vi "main.vi"() -> ()   [LabVIEW 2022 SP3]
uses:
  controls/State_control.ctl
  controls/Data.ctl
  <vilib>/Utility/TDMS File Viewer/NI_TDMS File Viewer.lvlib
panel:
  out "Current":dbl(graph)
  out "Voltage":dbl(graph)
  out "Current":dbl[](array[numeric])
  out "Voltage":dbl[](array[numeric])
  in  "Pocet prumer":i8 min=1 max=20 step=1
  out "Doba mereni [ms]":i16
  in  "Pocet vz":i32
  in  "vzorky/s":enum16{"Slow", "2F2F"}(ring)
  out "IDN commnad 4":string
  in  "GPD-3303S":refnum<visa-resource-name>
  in  "Stop":bool
  in  "Store data":bool
  in  "Reset array":bool
  in  "Start meas":bool
  out "IDN commnad":string
  in  "Agilent 34401A":refnum<visa-resource-name>
  in  "Agilent 34450A":refnum<visa-resource-name>
  out "IDN commnad 3":string
  out "State":T1=enum."SaveData"
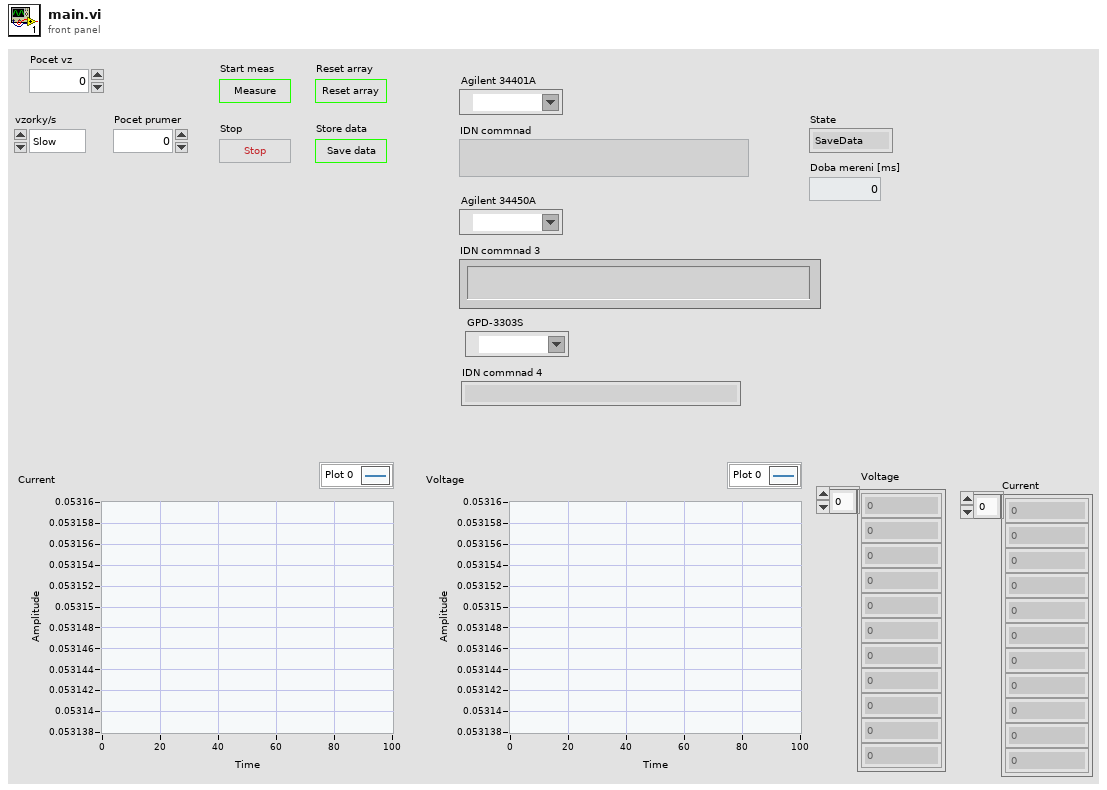
[diagram p1: front panel]
types:
  T1 = typedef "State_control.ctl" = enum16{"Init", "Waiting", "Measure", "SaveData", "Finish"}
  T2 = typedef "Data.ctl" = cluster{"No Sample":i32, "Samples/s":i32, "No to avg":i32, "Voltage":dbl[], "Current":dbl[], "Resistance":dbl[], "Temperature":dbl[], "Avg Voltage":dbl[], "Timestamp":timestamp[], "Avg Current":dbl[]}
  T3 = enum16{"open", "open or create", "create or replace", "create", "open (read-only)"}
  T4 = cluster{"Agilent 34401A":refnum<visa-resource-name>, "Agilent 34450A":refnum<visa-resource-name>}
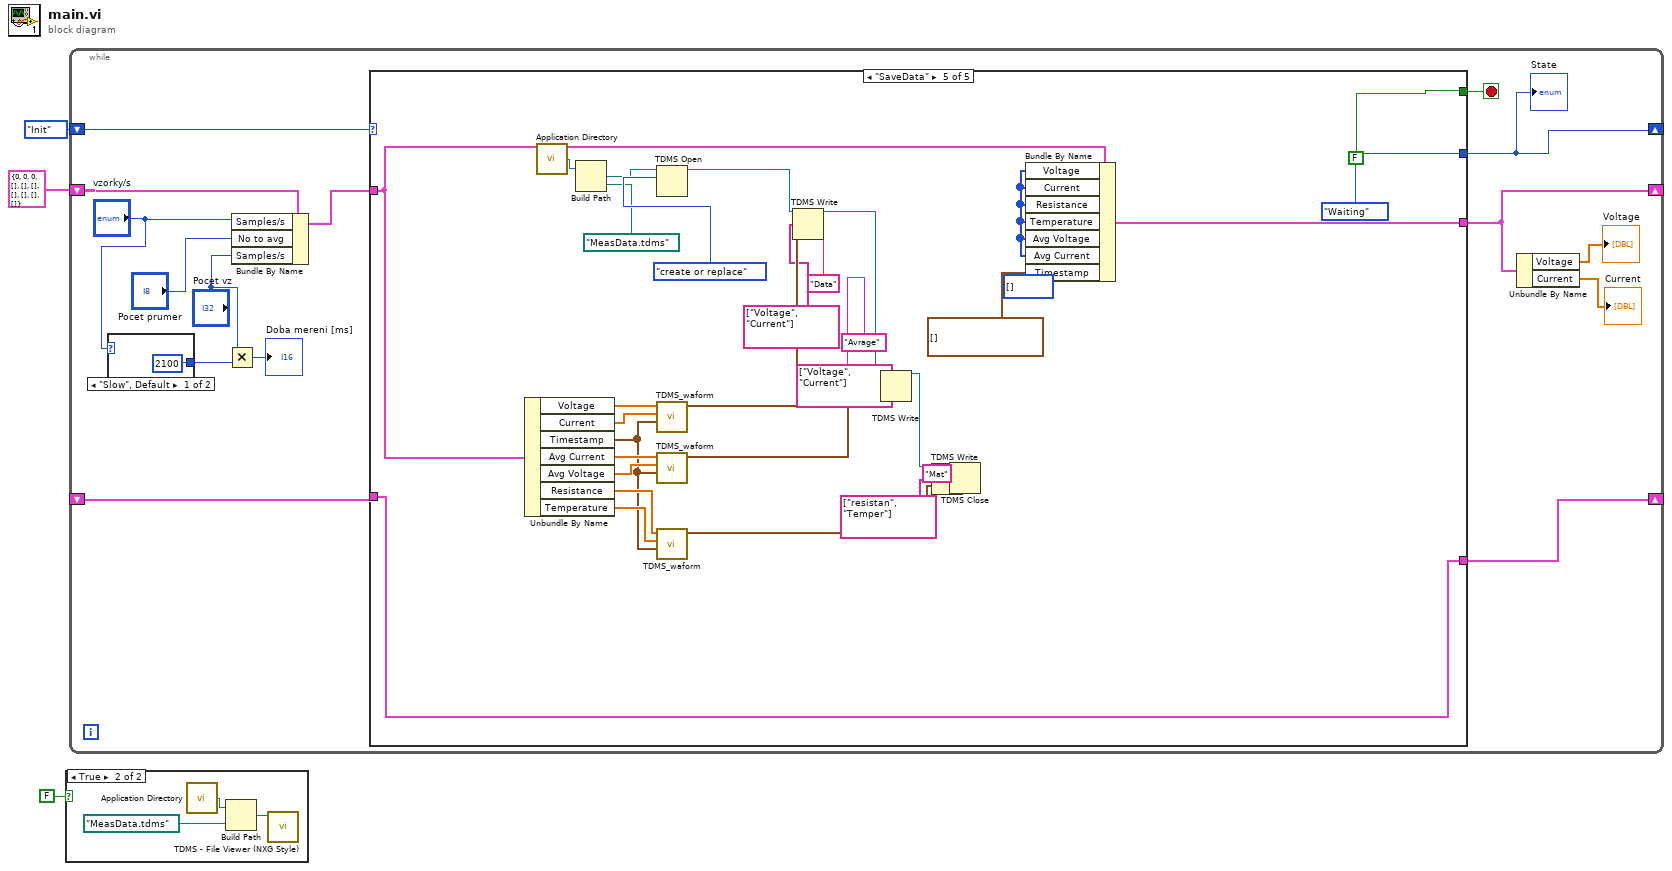
[diagram p0: block diagram]
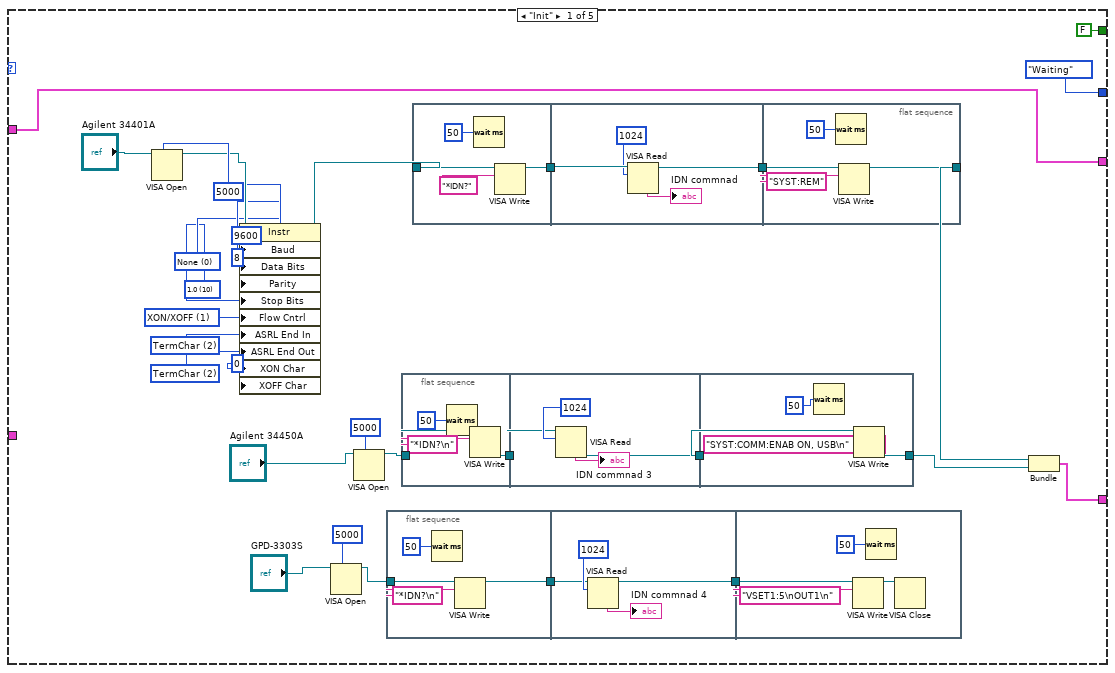
[diagram p2: hidden frame]
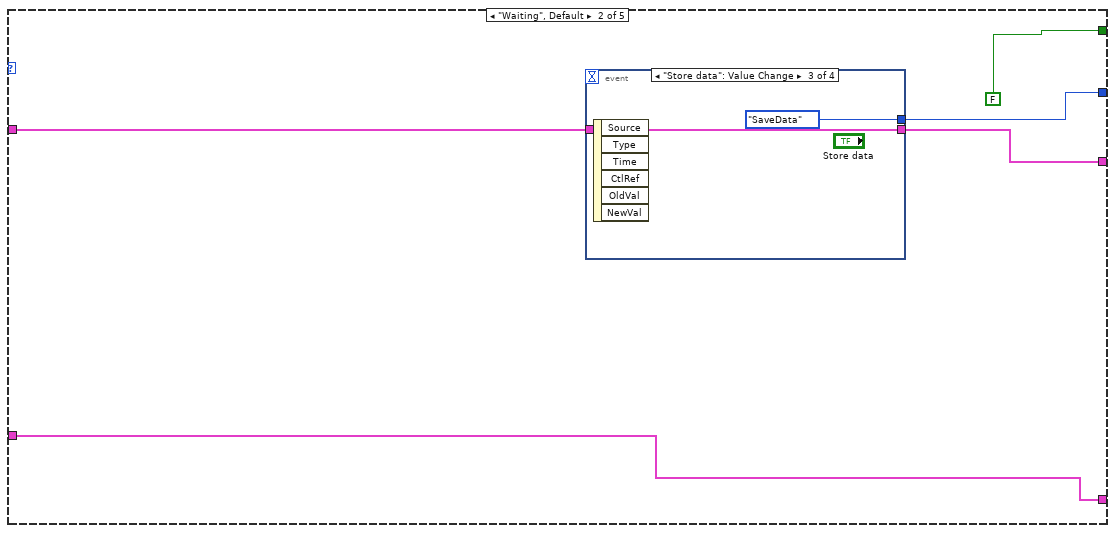
[diagram p3: hidden frame]
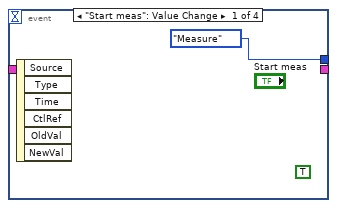
[diagram p4: hidden frame]
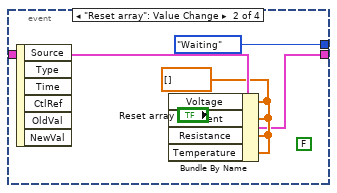
[diagram p5: hidden frame]
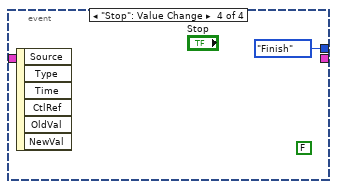
[diagram p6: hidden frame]
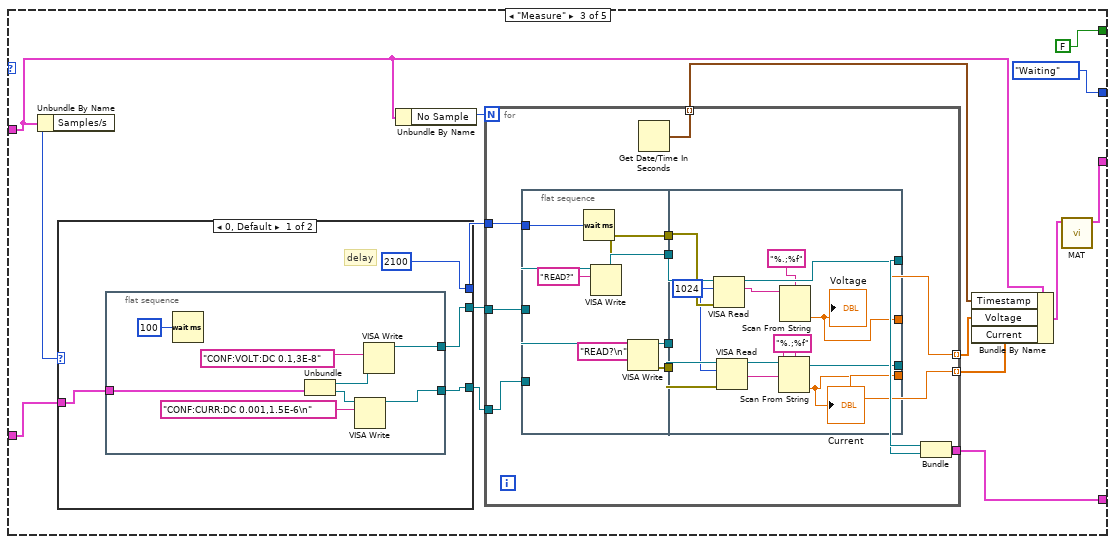
[diagram p7: hidden frame]
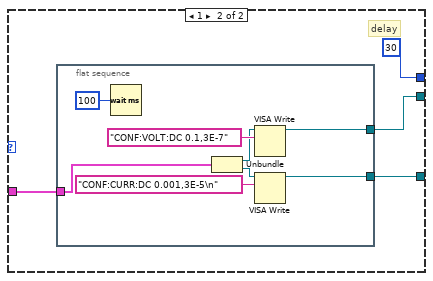
[diagram p8: hidden frame]
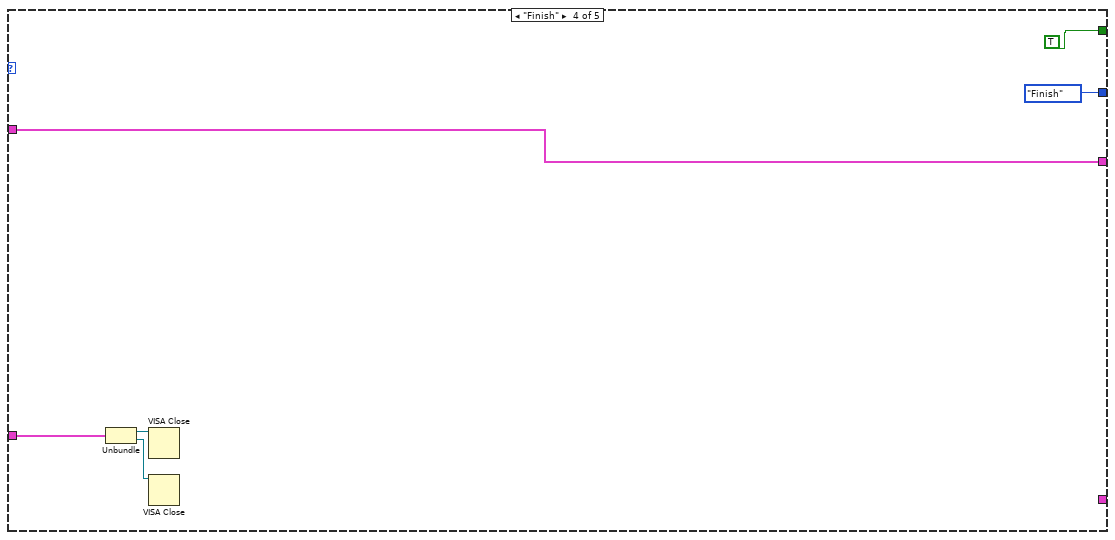
[diagram p9: hidden frame]
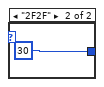
[diagram p10: hidden frame]
diagram:
  n1 = case shown="True" FALSE {
    frame False {
    }
    frame True {
      n2 = call <vilib>:"Application Directory.vi"() -> ("Application Directory"=w6:path)
      n3 = Build Path(base path=w6, name or relative path=path "MeasData.tdms") -> (appended path=w4:path)
      n4 = call <vilib>:"TDMS - File Viewer (NXG Style).vi"("file in"=w4) -> ()  [unwired: 9 in, 2 out]
    }
  }
  n5 = while {
    shift-right: [w17] -> _
    shift-left: State_control."Init" ("State") -> [w21]
    shift-right: [w14] -> _
    shift-left: T2 {"No Sample"=0, "Samples/s"=0, "No to avg"=0, "Voltage"=[], "Current"=[], "Resistance"=[], "Temperature"=[], "Avg Voltage"=[], "Timestamp"=[], "Avg Current"=[]} ("Data") -> [w16]
    shift-right: [w19] -> _
    shift-left: _ -> [w18]
    stop <- w20 stop-if-true
    n6 = case shown="\"Slow\", Default" "vzorky/s" {
      tunnel: [u32 2100 ("milliseconds to wait") u32 30 ("milliseconds to wait")] -> w10
      frame "Slow", Default {
      }
      frame "2F2F" {
      }
    }
    n7 = Multiply(x="Pocet vz", y=w10) -> (x*y=→"Doba mereni [ms]":u32)
    n8 = Bundle By Name(cluster=w16, "Samples/s"="vzorky/s", "No to avg"="Pocet prumer", "Samples/s"="Pocet vz") -> (w15:T2)
    n9 = case shown="\"SaveData\"" w21 {
      tunnel: [State_control."Waiting" ("State 2") w91 State_control."Waiting" ("State 2") State_control."Finish" ("State 2") State_control."Waiting" ("State 2")] -> w17
      tunnel: [FALSE FALSE FALSE TRUE FALSE] -> w20
      tunnel: w15 -> [w22 w90 w107 w176 w185]
      tunnel: [w22 w89 w106 w176 w184] -> w14
      tunnel: [w23 w92 w111 _ w208] -> w19
      tunnel: w18 -> [_ w92 w114 w179 w208]
      frame "Init" {
        w42 = u16 2 items=["None", "Last Bit", "TermChar", "Break"] ("Serial Settings:End Mode for Writes")
        w43 = u16 2 items=["None", "Last Bit", "TermChar"] ("Serial Settings:End Mode for Reads")
        w44 = u16 1 items=["None", "XON/XOFF", "RTS/CTS", "XON/XOFF & RTS/CTS", "DTR/DSR", "XON/XOFF & DTR/DSR"] ("Serial Settings:Flow Control")
        w45 = u16 10 items=["1.0"=10, "1.5"=15, "2.0"=20] ("Serial Settings:Stop Bits")
        w46 = u16 0 items=["None", "Odd", "Even", "Mark", "Space"] ("Serial Settings:Parity")
        n10 = VISA Open(timeout (0)=u32 5000 ("VISA Open timeout (0)"), VISA resource name="Agilent 34401A") -> (VISA resource name=w49:refnum<visa-resource-name>)  [unwired: 3 in, 1 out]
        n11 = property class="Instr"(reference=w49, "Baud"=u32 9600 ("Serial Settings:Baud Rate"), "Data Bits"=u16 8 ("Serial Settings:Data Bits"), "Parity"=w46, "Stop Bits"=w45, "Flow Cntrl"=w44, "ASRL End In"=w43, "ASRL End Out"=w42, "XON Char"=u8 0 ("Serial Settings:Flow Control XON Character"), "XOFF Char"=u8 0 ("Serial Settings:Flow Control XOFF Character")) -> (reference out=w38:refnum<visa-resource-name>)  [unwired: 1 in, 1 out]
        n12 = VISA Open(timeout (0)=u32 5000 ("VISA Open timeout (0)"), VISA resource name="GPD-3303S") -> (VISA resource name=w26:refnum<visa-resource-name>)  [unwired: 3 in, 1 out]
        n13 = VISA Open(timeout (0)=u32 5000 ("VISA Open timeout (0)"), VISA resource name="Agilent 34450A") -> (VISA resource name=w31:refnum<visa-resource-name>)  [unwired: 3 in, 1 out]
        n14 = flat-sequence {
          tunnel: [w55] -> w28
          tunnel: w26 -> [w53]
          tunnel: w28 -> [w59]
          tunnel: [w58] -> w27
          tunnel: w27 -> [w62]
          frame #0 {
            n15 = Wait (ms)(milliseconds to wait=u32 50) -> ()  [unwired: 1 out]
            n16 = VISA Write(VISA resource name=w53, write buffer="*IDN?\n") -> (VISA resource name out=w55:refnum<visa-resource-name>)  [unwired: 1 in, 2 out]
          }
          frame #1 {
            n17 = VISA Read(VISA resource name=w59, byte count=u32 1024) -> (VISA resource name out=w58:refnum<visa-resource-name>, read buffer=→"IDN commnad 4":string)  [unwired: 1 in, 2 out]
          }
          frame #2 {
            n18 = VISA Write(VISA resource name=w62, write buffer="VSET1:5\nOUT1\n") -> (VISA resource name out=w61:refnum<visa-resource-name>)  [unwired: 1 in, 2 out]
            n19 = Wait (ms)(milliseconds to wait=u32 50) -> ()  [unwired: 1 out]
            n20 = VISA Close(VISA resource name=w61) -> ()  [unwired: 1 in, 1 out]
          }
        }
        n21 = flat-sequence {
          tunnel: [w67] -> w35
          tunnel: w31 -> [w65]
          tunnel: w35 -> [w71]
          tunnel: [w70] -> w34
          tunnel: [w73] -> w24
          tunnel: w34 -> [w74]
          frame #0 {
            n22 = Wait (ms)(milliseconds to wait=u32 50) -> ()  [unwired: 1 out]
            n23 = VISA Write(VISA resource name=w65, write buffer="*IDN?\n") -> (VISA resource name out=w67:refnum<visa-resource-name>)  [unwired: 1 in, 2 out]
          }
          frame #1 {
            n24 = VISA Read(VISA resource name=w71, byte count=u32 1024) -> (VISA resource name out=w70:refnum<visa-resource-name>, read buffer=→"IDN commnad 3":string)  [unwired: 1 in, 2 out]
          }
          frame #2 {
            n25 = Wait (ms)(milliseconds to wait=u32 50) -> ()  [unwired: 1 out]
            n26 = VISA Write(VISA resource name=w74, write buffer="SYST:COMM:ENAB ON, USB\n") -> (VISA resource name out=w73:refnum<visa-resource-name>)  [unwired: 1 in, 2 out]
          }
        }
        n27 = flat-sequence {
          tunnel: w38 -> [w80]
          tunnel: [w78] -> w39
          tunnel: w39 -> [w84]
          tunnel: [w83] -> w37
          tunnel: [w86] -> w25
          tunnel: w37 -> [w87]
          frame #0 {
            n28 = Wait (ms)(milliseconds to wait=u32 50) -> ()  [unwired: 1 out]
            n29 = VISA Write(VISA resource name=w80, write buffer="*IDN?") -> (VISA resource name out=w78:refnum<visa-resource-name>)  [unwired: 1 in, 2 out]
          }
          frame #1 {
            n30 = VISA Read(VISA resource name=w84, byte count=u32 1024) -> (VISA resource name out=w83:refnum<visa-resource-name>, read buffer=→"IDN commnad":string)  [unwired: 1 in, 2 out]
          }
          frame #2 {
            n31 = Wait (ms)(milliseconds to wait=u32 50) -> ()  [unwired: 1 out]
            n32 = VISA Write(VISA resource name=w87, write buffer="SYST:REM") -> (VISA resource name out=w86:refnum<visa-resource-name>)  [unwired: 1 in, 2 out]
          }
        }
        n33 = Bundle("Agilent 34401A"=w25, "Agilent 34450A"=w24) -> (w23:T4)  [unwired: 1 in]
      }
      frame "Waiting", Default {
        n34 = event shown="[2] \"Store data\": Value Change" {
          selector: _ -> [_ _ _ _]
          dyn-events: _ -> [_ _ _ _]
          timeout: _ -> [_ _ _ _]
          tunnel: [State_control."Measure" ("State 2") State_control."Waiting" ("State 2") State_control."SaveData" ("State 2") State_control."Finish" ("State 2")] -> w91
          tunnel: w90 -> [_ w97 w99 _]
          tunnel: [_ w95 w99 _] -> w89
          event "Start meas": Value Change {
            (unwired) TRUE
            n35 = event-data() -> ()  [unwired: 1 in, 6 out]
          }
          event "Reset array": Value Change {
            w96 = dbl[] [] ("Voltage")
            (unwired) FALSE
            n36 = event-data() -> ()  [unwired: 1 in, 6 out]
            n37 = Bundle By Name(cluster=w97, "Voltage"=w96, "Current"=w96, "Resistance"=w96, "Temperature"=w96) -> (w95:T2)
          }
          event "Store data": Value Change {
            n38 = event-data() -> ()  [unwired: 1 in, 6 out]
          }
          event "Stop": Value Change {
            (unwired) FALSE
            n39 = event-data() -> ()  [unwired: 1 in, 6 out]
          }
        }
      }
      frame "Measure" {
        n40 = Unbundle By Name(w107) -> ("Samples/s"=w108:i32)
        n41 = case shown="0, Default" w108 {
          tunnel: w114 -> [w155 w167]
          tunnel: [w152 w166] -> w113
          tunnel: [w153 w165] -> w112
          tunnel: [u32 2100 ("milliseconds to wait") u32 30 ("milliseconds to wait")] -> w110
          frame 0, Default {
            # "delay"
            n42 = flat-sequence {
              tunnel: [w161] -> w153
              tunnel: w155 -> [w158]
              tunnel: [w160] -> w152
              frame #0 {
                n43 = Wait (ms)(milliseconds to wait=u32 100) -> ()  [unwired: 1 out]
                n44 = Unbundle(w158) -> ("Agilent 34401A"=w157:refnum<visa-resource-name>, "Agilent 34450A"=w156:refnum<visa-resource-name>)
                n45 = VISA Write(VISA resource name=w156, write buffer="CONF:CURR:DC 0.001,1.5E-6\n") -> (VISA resource name out=w160:refnum<visa-resource-name>)  [unwired: 1 in, 2 out]
                n46 = VISA Write(VISA resource name=w157, write buffer="CONF:VOLT:DC 0.1,3E-8") -> (VISA resource name out=w161:refnum<visa-resource-name>)  [unwired: 1 in, 2 out]
              }
            }
          }
          frame 1 {
            # "delay"
            n47 = flat-sequence {
              tunnel: [w173] -> w165
              tunnel: w167 -> [w170]
              tunnel: [w172] -> w166
              frame #0 {
                n48 = Wait (ms)(milliseconds to wait=u32 100) -> ()  [unwired: 1 out]
                n49 = Unbundle(w170) -> ("Agilent 34401A"=w169:refnum<visa-resource-name>, "Agilent 34450A"=w168:refnum<visa-resource-name>)
                n50 = VISA Write(VISA resource name=w169, write buffer="CONF:VOLT:DC 0.1,3E-7") -> (VISA resource name out=w173:refnum<visa-resource-name>)  [unwired: 1 in, 2 out]
                n51 = VISA Write(VISA resource name=w168, write buffer="CONF:CURR:DC 0.001,3E-5\n") -> (VISA resource name out=w172:refnum<visa-resource-name>)  [unwired: 1 in, 2 out]
              }
            }
          }
        }
        n52 = Unbundle By Name(w107) -> ("No Sample"=w109:i32)
        n53 = for {
          N: w109 -> [_]
          tunnel: w113 -> [w125]
          tunnel: w112 -> [w124]
          tunnel: [w121] -> w111
          tunnel: w110 -> [w120]
          tunnel: [w118] -> w102 mode=indexing
          tunnel: [w117] -> w103 mode=indexing
          tunnel: [w119] -> w105 mode=indexing
          n54 = flat-sequence {
            tunnel: [w138] -> w129
            tunnel: w124 -> [w137]
            tunnel: [w136] -> w128
            tunnel: w125 -> [w135]
            tunnel: [w134] -> w127
            tunnel: [w133] -> w126
            tunnel: w120 -> [w130]
            tunnel: w129 -> [w150]
            tunnel: [w151] -> w123
            tunnel: w128 -> [w149]
            tunnel: w127 -> [w148]
            tunnel: w126 -> [w147]
            tunnel: [w146] -> w122
            tunnel: [w143] -> w118
            tunnel: [w141] -> w117
            frame #0 {
              n55 = Wait (ms)(milliseconds to wait=w130) -> ()  [unwired: 1 out]
              n56 = VISA Write(VISA resource name=w137, write buffer="READ?") -> (VISA resource name out=w138:refnum<visa-resource-name>, error out=w136:errorcluster)  [unwired: 1 in, 1 out]
              n57 = VISA Write(VISA resource name=w135, write buffer="READ?\n") -> (VISA resource name out=w133:refnum<visa-resource-name>, error out=w134:errorcluster)  [unwired: 1 in, 1 out]
            }
            frame #1 {
              w145 = u32 1024 ("byte count")
              n58 = VISA Read(VISA resource name=w150, byte count=w145, error in (no error)=w149) -> (VISA resource name out=w151:refnum<visa-resource-name>, read buffer=w144:string)  [unwired: 2 out]
              n59 = VISA Read(VISA resource name=w147, byte count=w145, error in (no error)=w148) -> (VISA resource name out=w146:refnum<visa-resource-name>, read buffer=w142:string)  [unwired: 2 out]
              n60 = Scan From String(format string="%.;%f", input string=w142) -> (output 1=w141:dbl)  [unwired: 3 in, 3 out]
              "Current" <- w141
              n61 = Scan From String(format string="%.;%f", input string=w144) -> (output 1=w143:dbl)  [unwired: 3 in, 3 out]
              "Voltage" <- w143
            }
          }
          n62 = Get Date/Time In Seconds() -> (seconds since 1Jan1904=w119:timestamp)
          n63 = Bundle("Agilent 34401A"=w123, "Agilent 34450A"=w122) -> (w121:T4)  [unwired: 1 in]
        }
        n64 = Bundle By Name(cluster=w107, "Timestamp"=w105, "Voltage"=w102, "Current"=w103) -> (w104:T2)
        n65 = call "MAT.vi"("Data in"=w104) -> ("Data out"=w106:T2)  [unwired: 10 in]
      }
      frame "Finish" {
        n66 = Unbundle(w179) -> ("Agilent 34401A"=w178:refnum<visa-resource-name>, "Agilent 34450A"=w177:refnum<visa-resource-name>)
        n67 = VISA Close(VISA resource name=w178) -> ()  [unwired: 1 in, 1 out]
        n68 = VISA Close(VISA resource name=w177) -> ()  [unwired: 1 in, 1 out]
      }
      frame "SaveData" {
        w183 = i32[] []
        n69 = Unbundle By Name(w185) -> ("Voltage"=w203:dbl[], "Current"=w207:dbl[], "Timestamp"=w191:timestamp[], "Avg Current"=w196:dbl[], "Avg Voltage"=w195:dbl[], "Resistance"=w193:dbl[], "Temperature"=w192:dbl[])
        n70 = call <vilib>:"Application Directory.vi"() -> ("Application Directory"=w206:path)
        n71 = Build Path(base path=w206, name or relative path=path "MeasData.tdms") -> (appended path=w205:path)
        n72 = TDMS Open(10:T3."create or replace" ("operation (0:open)"), 11:w205) -> (3:w209:refnum<k34>)  [unwired: 5 in, 1 out]
        n73 = call "TDMS_waform.vi"("Timestamp"=w191, "Current"=w207, "Voltage"=w203) -> ("Array"=w202:waveform(dbl)[])  [unwired: 8 in]
        n74 = call "TDMS_waform.vi"("Timestamp"=w191, "Current"=w195, "Voltage"=w196) -> ("Array"=w194:waveform(dbl)[])  [unwired: 8 in]
        n75 = call "TDMS_waform.vi"("Timestamp"=w191, "Current"=w192, "Voltage"=w193) -> ("Array"=w186:waveform(dbl)[])  [unwired: 8 in]
        n76 = TDMS Write(0:w209, 5:"Data" ("group name in (Untitled)"), 7:string[] ["Voltage", "Current"], 9:w202) -> (4:w199:refnum<k34>)  [unwired: 2 in, 3 out]
        n77 = TDMS Write(0:w199, 5:"Avrage" ("group name in (Untitled)"), 7:string[] ["Voltage", "Current"], 9:w194) -> (4:w187:refnum<k34>)  [unwired: 2 in, 3 out]
        n78 = TDMS Write(0:w187, 5:"Mat" ("group name in (Untitled)"), 7:string[] ["resistan", "Temper"], 9:w186) -> (4:w188:refnum<k34>)  [unwired: 2 in, 3 out]
        n79 = TDMS Close(11:w188) -> ()  [unwired: 1 in, 2 out]
        n80 = Bundle By Name(cluster=w185, "Voltage"=w183, "Current"=w183, "Resistance"=w183, "Temperature"=w183, "Avg Voltage"=w183, "Avg Current"=w183, "Timestamp"=timestamp[] []) -> (w184:T2)
      }
    }
    "State" <- w17
    n81 = Unbundle By Name(w14) -> ("Voltage"=→"Voltage":dbl[], "Current"=→"Current":dbl[])
  }
